vi "main.vi"() -> ()   [LabVIEW 2023]
uses:
  CONTROLS/states.ctl
panel:
  out "Meldung":string
  out "Enum":T1
  in  "stop":bool
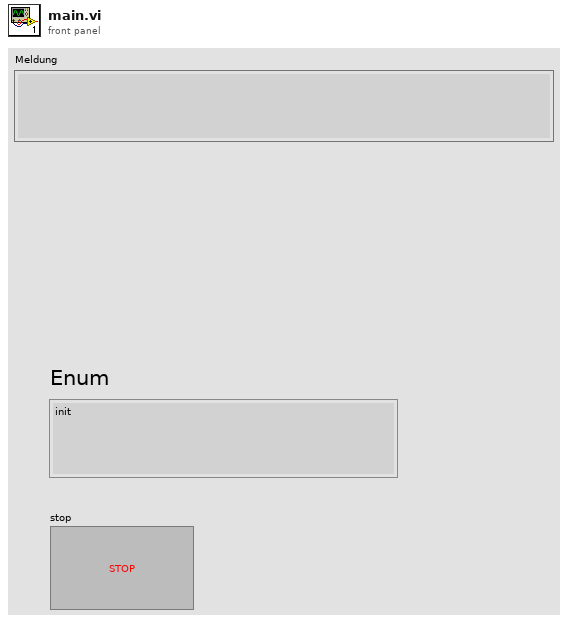
[diagram p1: front panel]
types:
  T1 = typedef "states.ctl" = enum16{"init", "read", "write", "Kundeneingabe", "Betonauswahl", "Bezahlprozeß", "Rechnung", "Zudaten mit Gewichtmessung", "Stop"}
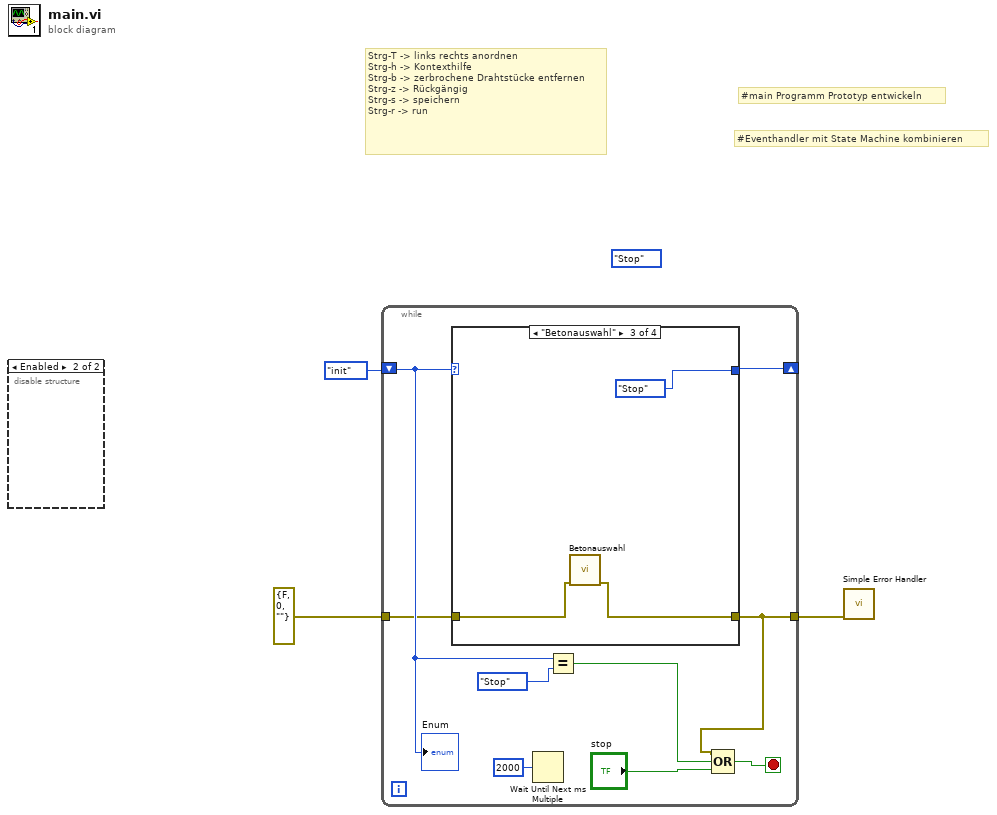
[diagram p0: block diagram]
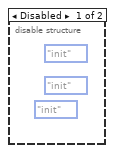
[diagram p2: hidden frame]
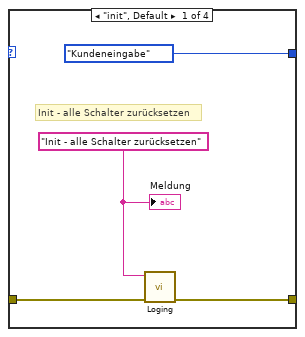
[diagram p3: hidden frame]
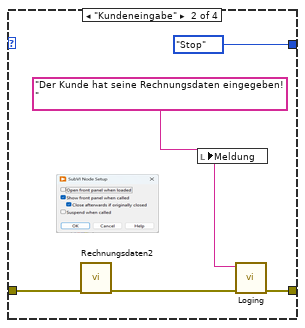
[diagram p4: hidden frame]
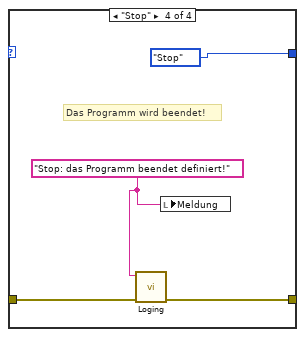
[diagram p5: hidden frame]
diagram:
  (unwired) states."Stop"
  # "#Eventhandler mit State Machine kombinieren"
  # "#main Programm Prototyp entwickeln"
  # "Strg-T -> links rechts anordnen\nStrg-h -> Kontexthilfe\nStrg-b -> zerbrochene Drahtstücke entfernen\nStrg-z -> Rückgängig\nStrg-s -> speichern\nStrg-r -> run"
  n1 = disable-structure shown="Enabled" {
    frame Disabled {
      (unwired) states."init"
      (unwired) states."init"
      (unwired) states."init"
    }
    frame Enabled {
    }
  }
  n2 = while {
    shift-right: [w12] -> _
    shift-left: states."init" -> [w10]
    tunnel: errorcluster {"status"=FALSE, "code"=0, "source"=""} ("error in") -> [w5]
    tunnel: [w4] -> w2
    stop <- w7 stop-if-true
    n3 = case shown="\"Betonauswahl\"" w10 {
      tunnel: [states."Kundeneingabe" states."Stop" states."Stop" states."Stop"] -> w12
      tunnel: w5 -> [w14 w18 w22 w26]
      tunnel: [w13 w19 w23 w25] -> w4
      frame "init", Default {
        w15 = "Init - alle Schalter zurücksetzen" ("Meldung")
        # "Init - alle Schalter zurücksetzen"
        n4 = call "Loging.vi"("error in"=w14, "log"=w15) -> ("error out"=w13:errorcluster)  [unwired: 9 in]
        "Meldung" <- w15
      }
      frame "Kundeneingabe" {
        w20 = "Der Kunde hat seine Rechnungsdaten eingegeben!   " ("Meldung")
        n5 = call "Rechnungsdaten2.vi"("error in (no error)"=w18) -> ("error out"=w17:errorcluster)  [unwired: 10 in]
        n6 = local write "Meldung"(w20) -> ()
        n7 = call "Loging.vi"("error in"=w17, "log"=w20) -> ("error out"=w19:errorcluster)  [unwired: 9 in]
      }
      frame "Betonauswahl" {
        n8 = call "Betonauswahl.vi"("error in (no error)"=w22) -> ("error out"=w23:errorcluster)  [unwired: 10 in]
      }
      frame "Stop" {
        w27 = "Stop: das Programm beendet definiert!" ("Meldung")
        # "Das Programm wird beendet!"
        n9 = call "Loging.vi"("error in"=w26, "log"=w27) -> ("error out"=w25:errorcluster)  [unwired: 9 in]
        n10 = local write "Meldung"(w27) -> ()
      }
    }
    n11 = Wait Until Next ms Multiple(millisecond multiple=u32 2000) -> ()  [unwired: 1 out]
    n12 = Equal?(x=w10, y=states."Stop") -> (x = y?=w9:bool)
    n13 = Compound Arithmetic op=OR(w4, w9, "stop") -> (w7:bool)
    "Enum" <- w10
  }
  n14 = call <vilib>:"Simple Error Handler.vi"("error in (no error)"=w2) -> ()  [unwired: 4 in, 5 out]
